vi "Calculate pivotal X.vi"(8 "error in (no error)":errorcluster, 11 "Tomo in":refnum<class "Tomo.lvclass">) -> (0 "error out":errorcluster, 3 "Tomo out":refnum<class "Tomo.lvclass">)   [LabVIEW 2012, in "Tomo.lvclass"]
uses:
  Tomo.lvclass
  Tomo.lvclass/Tomo.ctl
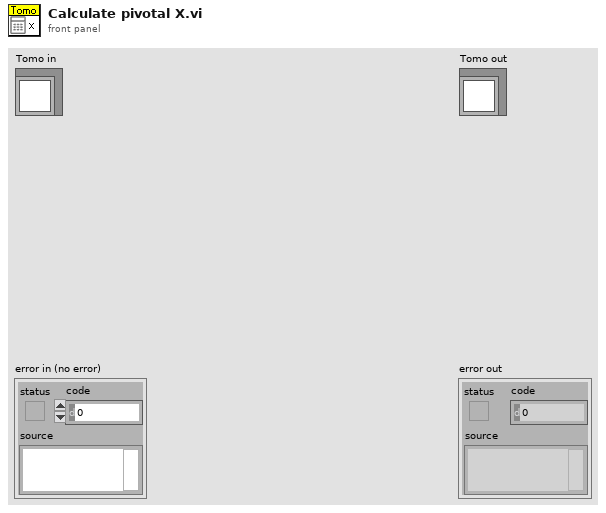
[diagram p1: front panel]
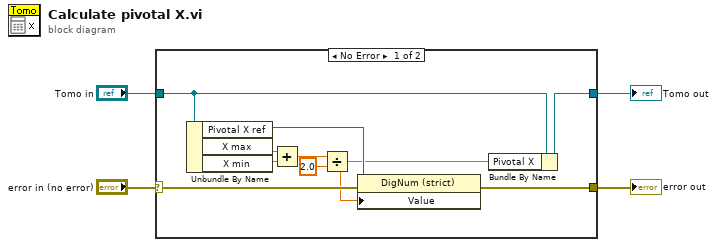
[diagram p0: block diagram]
diagram:
  n1 = case shown="No Error" "error in (no error)" {
    selector: "error in (no error)" -> [w9 w16]
    tunnel: [w8 w16] -> w3
    tunnel: [w6 w15] -> w1
    tunnel: "Tomo in" -> [w7 w15]
    frame No Error {
      n2 = Unbundle By Name(w7) -> ("Pivotal X ref"=w10:refnum<vi>, "X max"=w14:dbl[unit], "X min"=w13:dbl[unit])
      n3 = Add(x=w14, y=w13) -> (x+y=w12:dbl[unit])
      n4 = Divide(x=w12, y=2.0) -> (x/y=w5:dbl[unit])
      n5 = property class="DigNum (strict)"(reference=w10, error in=w9, "Value"=w5) -> (error out=w8:errorcluster)  [unwired: 1 out]
      n6 = Bundle By Name(cluster=w7, "Pivotal X"=w5) -> (w6:refnum<class "Tomo.lvclass">)
    }
    frame Error {
    }
  }
  "error out" <- w3
  "Tomo out" <- w1
